vi "Test JSON Variant Tools.vi"() -> ()   [LabVIEW 2013]
doc: "Demonstrates the use of the Variant JSON VIs for converting to and from a complex cluster."
uses:
  json-api-labview/JSON Scalar/Infinity&NaN.ctl
  json-api-labview/JSON Value/JSON Value.lvclass
  json-api-labview/JSON Value/Set from JSON string.vi
  json-api-labview/Variant JSON/Get as Variant.vi
  json-api-labview/Variant JSON/Variant to JSON.vi
  json-api-labview/Get Polymorphic/JSON GetSet.lvlib
  json-api-labview/Variant JSON/Variant JSON.lvlib
  JSON2.lvlib
  json-api-labview/support/JSON support.lvlib
panel:
  in  "Pretty Print?":bool=TRUE
  out "Var to JSON":dbl format="%#_4p"
  in  "Direct":bool
  out "Total Times":dbl[](array[numeric]) format="%#_4p"
  out "to Variant":dbl format="%#_4p"
  out "from JSON":dbl format="%#_4p"
  out "to JSON":dbl format="%#_4p"
  out "Set Var":dbl format="%#_4p"
  out "length":i32
  in  "Treatment of Infinity/NaN":T1
  out "error out":errorcluster
  out "Variant after setting":variant
  out "Cluster after setting":T2={"T1"=0.0, "Nest"={"NestNest"={"A"="", "Complex"=0.0+0.0i, "C"=0.0}, "Enum"=enum."AAA"}, "Test Array"=[], "Boolean 1"=FALSE, "T2"="", "Boolean 2"=FALSE, "Time Stamp"=timestamp(0 s since 1904-01-01), "Infinity"=0.0, "NAN"=0.0, "<JSON>EmbededJSON"="", "waveform"={"t0"=timestamp(0 s since 1904-01-01), "dt"=1.0, "Y"=[]}, "Test Array 2D"=[], "String Array"=[["", "", ""]], "Path"=path "", "Unnamed Cluster"={"Goes to Array", 2.0, "<JSON>"="{\"a\"=1234}"}}
  in  "Creation cluster":T3={"T2"="Test \"quote\",\nand newline.", "Nest"={"Enum"=enum."CCC (with a space)", "NestNest"={"A"=34.0, "Complex"=2.0+3.1i, "C"="1.23 string"}}, "Test Array"=array[1001 elements], "Boolean 1"=TRUE, "T1"=456.78900146484375, "Boolean 2"="true (a string)", "Time Stamp"=timestamp(3434102896.3125 s since 1904-01-01), "Extra item"="test2", "Infinity"=inf, "NAN"=nan, "<JSON>EmbededJSON"="{\"t\":123}", "waveform"={"t0"=timestamp(3436250625 s since 1904-01-01), "dt"=1.0, "Y"=[23.0, 34.0]}, "Test Array 2D"=array22x22[484 elements], "String Array"=[["one", "number 2", "three"], ["1one", "two", "3"]], "Unnamed Cluster"={"Cluster to Array", 2.0, "<JSON>"="{\"a\":1234}"}, "Path"=path "c:/temp123.txt", "Variant"=variant} {"Test Array" format="%#_19g"}
  out "JSON String created":string
  # "see diagram"
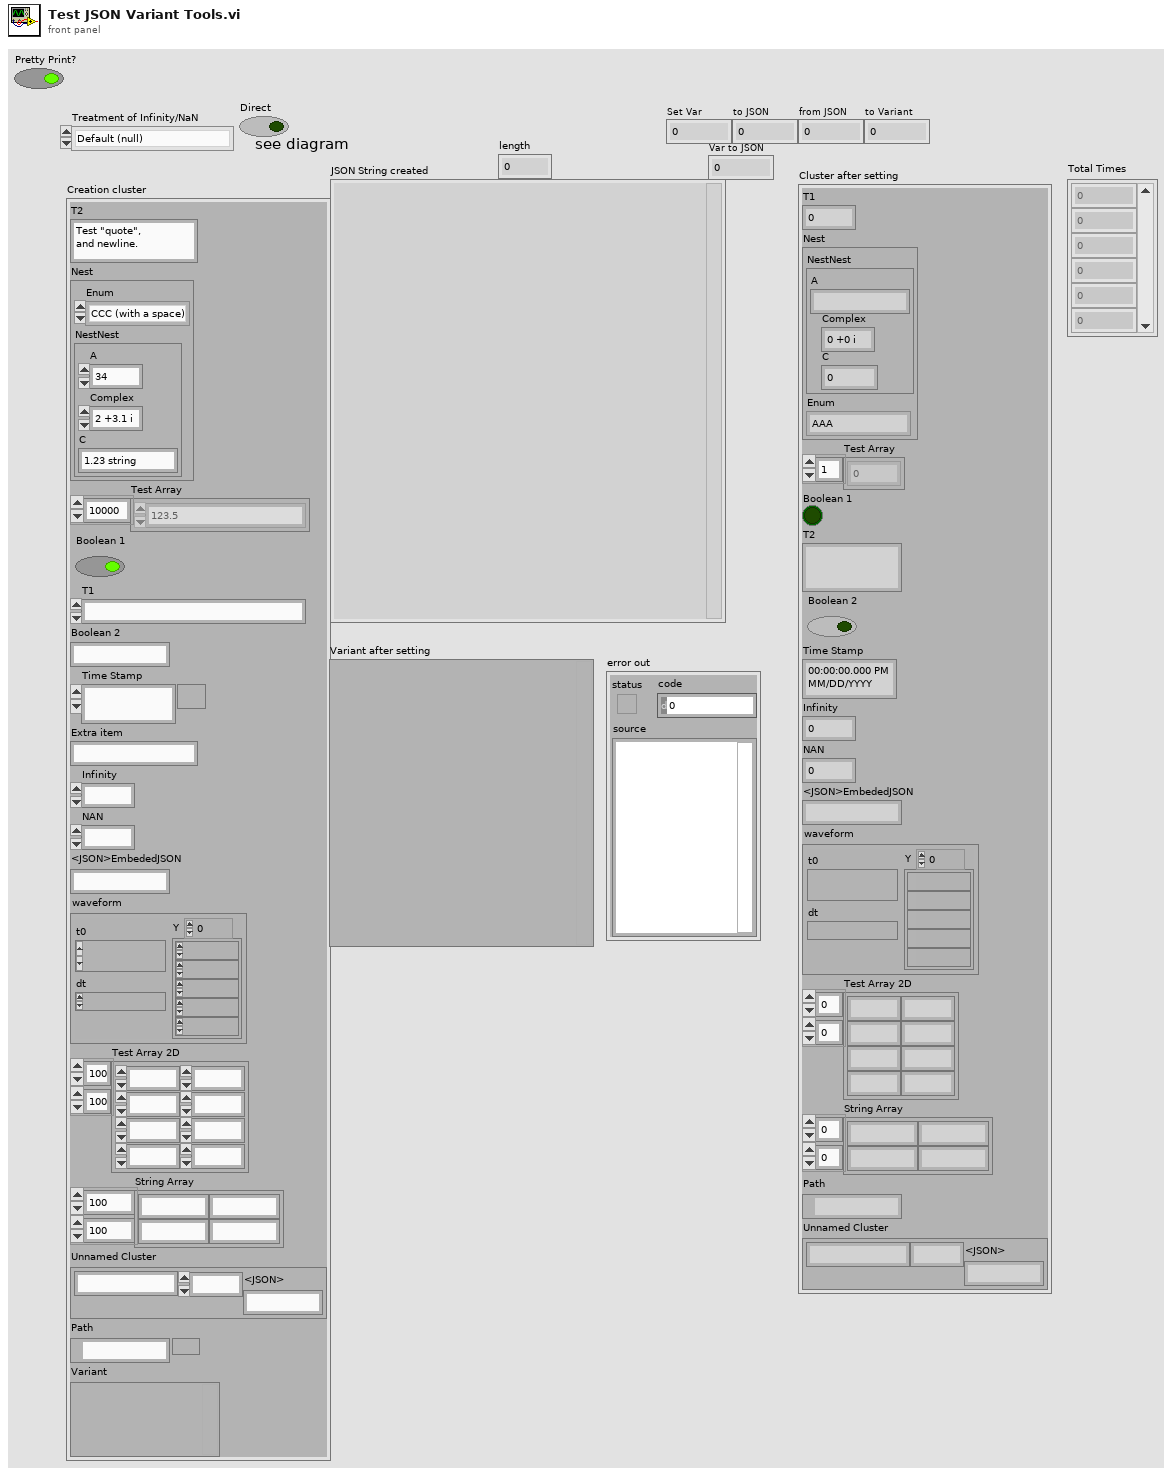
[diagram p1: front panel]
types:
  T1 = typedef "JSON support.lvlib/Infinity&NaN.ctl" = enum16{"Default (null)", "Extended", "LabVIEW extensions"}
  T2 = cluster{"T1":dbl, "Nest":cluster{"NestNest":cluster{"A":string, "Complex":cdb, "C":dbl}, "Enum":enum16{"AAA", "BBB", "CCC (with a space)"}}, "Test Array":dbl[], "Boolean 1":bool, "T2":string, "Boolean 2":bool, "Time Stamp":timestamp, "Infinity":dbl, "NAN":dbl, "<JSON>EmbededJSON":string, "waveform":waveform(dbl), "Test Array 2D":dbl[][], "String Array":string[][], "Path":path, "Unnamed Cluster":cluster{string, dbl, "<JSON>":string}}
  T3 = cluster{"T2":string, "Nest":cluster{"Enum":enum16{"AAA", "BBB", "CCC (with a space)"}, "NestNest":cluster{"A":dbl, "Complex":cdb, "C":string}}, "Test Array":dbl[], "Boolean 1":bool, "T1":ext, "Boolean 2":string, "Time Stamp":timestamp, "Extra item":string, "Infinity":dbl, "NAN":dbl, "<JSON>EmbededJSON":string, "waveform":waveform(dbl), "Test Array 2D":dbl[][], "String Array":string[][], "Unnamed Cluster":cluster{string, dbl, "<JSON>":string}, "Path":path, "Variant":variant}
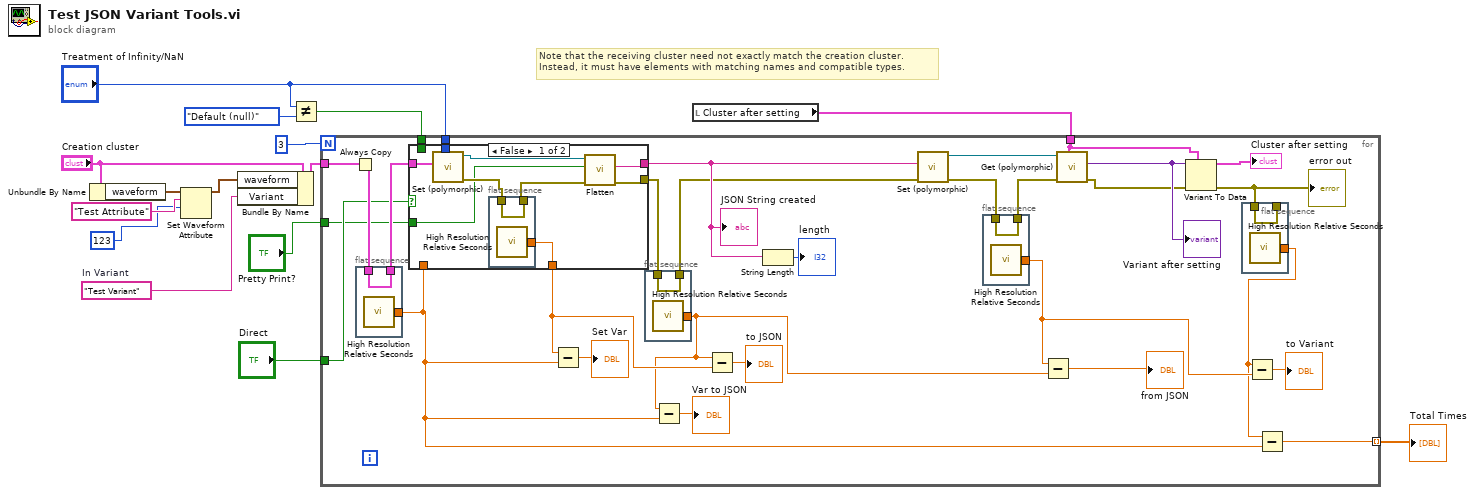
[diagram p0: block diagram]
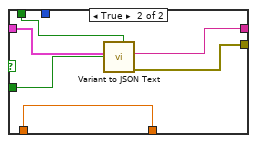
[diagram p2: hidden frame]
diagram:
  w2 = "Test Variant"  # In Variant
  # "Note that the receiving cluster need not exactly match the creation cluster.\nInstead, it must have elements with matching names and compatible types."
  n1 = Unbundle By Name("Creation cluster") -> ("waveform"=w11:waveform(dbl))
  n2 = Set Waveform Attribute(5:123, 6:"Test Attribute" ("name"), 7:w11) -> (3:w9:waveform(dbl))  [unwired: 1 in, 2 out]
  n3 = Bundle By Name(cluster="Creation cluster", "waveform"=w9, "Variant"=w2) -> (w10:T3)
  n4 = Not Equal?(x="Treatment of Infinity/NaN", y=Infinity&NaN."Default (null)") -> (x != y?=w3:bool)
  n5 = local read "Cluster after setting"() -> (w6:T2)
  n6 = for {
    N: 3 -> [_]
    tunnel: w10 -> [w33]
    tunnel: w6 -> [w41]
    tunnel: "Treatment of Infinity/NaN" -> [w40]
    tunnel: [w22] -> w14 mode=indexing
    tunnel: "Direct" -> [w21]
    tunnel: w3 -> [w17]
    tunnel: "Pretty Print?" -> [w16]
    n7 = Always Copy(1:w33) -> (0:w31:T3)
    n8 = flat-sequence {
      tunnel: [w66] -> w32
      tunnel: w31 -> [w66]
      tunnel: [w65] -> w18
      frame #0 {
        n9 = call <vilib>:"High Resolution Relative Seconds.vi"() -> ("relative seconds"=w65:dbl)
      }
    }
    n10 = case shown="False" w21 {
      tunnel: w40 -> [w54 _]
      tunnel: [w49 w61] -> w39
      tunnel: [w48 w60] -> w38
      tunnel: w32 -> [w52 w62]
      tunnel: [w51 w59] -> w28
      tunnel: w18 -> [_ w59]
      tunnel: w17 -> [_ w58]
      tunnel: w16 -> [w46 w57]
      frame False {
        n11 = call-poly "Set (polymorphic).vi"("Treatment of Infinity/NaN"=w54, "Variant"=w52) -> ("error out"=w53:errorcluster, "JSON Value out"=w50:refnum<class "JSON Value.lvclass">)  [unwired: 8 in]
        n12 = flat-sequence {
          tunnel: [w56] -> w47
          tunnel: w53 -> [w56]
          tunnel: [w55] -> w51
          frame #0 {
            n13 = call <vilib>:"High Resolution Relative Seconds.vi"() -> ("relative seconds"=w55:dbl)
          }
        }
        n14 = call-dynamic "Flatten.vi"("error in (no error)"=w47, "Pretty Print?"=w46, "JSON Value in"=w50) -> ("error out"=w48:errorcluster, "<JSON>"=w49:string)  [unwired: 7 in]
      }
      frame True {
        n15 = call "Variant to JSON Text.vi"("enable LabVIEW extensions? (T)"=w58, "Pretty Print?"=w57, "Variant"=w62) -> ("error out"=w60:errorcluster, "<JSON>"=w61:string)  [unwired: 7 in]
      }
    }
    "JSON String created" <- w39
    n16 = Subtract(x=w28, y=w18) -> (x-y=→"Set Var":dbl)
    n17 = flat-sequence {
      tunnel: w38 -> [w70]
      tunnel: [w70] -> w37
      tunnel: [w69] -> w19
      frame #0 {
        n18 = call <vilib>:"High Resolution Relative Seconds.vi"() -> ("relative seconds"=w69:dbl)
      }
    }
    n19 = Subtract(x=w19, y=w18) -> (x-y=→"Var to JSON":dbl)
    n20 = Subtract(x=w19, y=w28) -> (x-y=→"to JSON":dbl)
    n21 = String Length(string=w39) -> (length=→"length":i32)
    n22 = call-poly "Set (polymorphic).vi"("error in (no error)"=w37, "JSON stream"=w39) -> ("error out"=w35:errorcluster, "JSON Value out"=w42:refnum<class "JSON Value.lvclass">)  [unwired: 7 in, 1 out]
    n23 = flat-sequence {
      tunnel: w35 -> [w68]
      tunnel: [w68] -> w34
      tunnel: [w67] -> w24
      frame #0 {
        n24 = call <vilib>:"High Resolution Relative Seconds.vi"() -> ("relative seconds"=w67:dbl)
      }
    }
    n25 = Subtract(x=w24, y=w19) -> (x-y=→"from JSON":dbl)
    n26 = call-poly "Get (polymorphic).vi"("Variant (Data Type)"=w41, "error in (no error)"=w34, "JSON in"=w42) -> ("error out"=w43:errorcluster, "Variant out"=w45:variant)  [unwired: 6 in, 1 out]
    "Variant after setting" <- w45
    n27 = Variant To Data(error in=w43, type=w41, Variant=w45) -> (data=→"Cluster after setting":T2, error out=w25:errorcluster)
    "error out" <- w25
    n28 = flat-sequence {
      tunnel: w25 -> [w64]
      tunnel: [w64] -> _
      tunnel: [w63] -> w23
      frame #0 {
        n29 = call <vilib>:"High Resolution Relative Seconds.vi"() -> ("relative seconds"=w63:dbl)
      }
    }
    n30 = Subtract(x=w23, y=w24) -> (x-y=→"to Variant":dbl)
    n31 = Subtract(x=w23, y=w18) -> (x-y=w22:dbl)
  }
  "Total Times" <- w14
